vi "Utility Timestamp.vi"() -> (3 "Timestamp String":string)   [LabVIEW 2015]
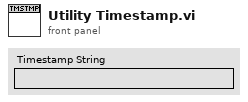
[diagram p1: front panel]
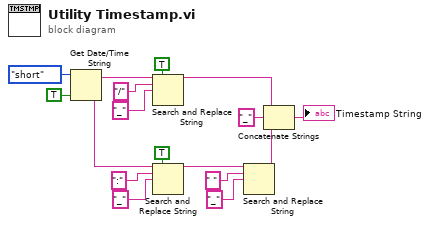
[diagram p0: block diagram]
diagram:
  n1 = Get Date/Time String(date format (0)=enum16{"short", "long", "abbreviated"}."short", want seconds? (F)=TRUE) -> (date string=w15:string, time string=w2:string)  [unwired: 1 in]
  n2 = Search and Replace String(replace all?=TRUE ("replace all? (F)"), input string=w15, search string="/", replace string="_" ("replace string (\"\")")) -> (result string=w1:string)  [unwired: 4 in, 3 out]
  n3 = Search and Replace String(replace all?=TRUE ("replace all? (F)"), input string=w2, search string=":", replace string="_" ("replace string (\"\")")) -> (result string=w6:string)  [unwired: 4 in, 3 out]
  n4 = Search and Replace String(input string=w6, search string=" ", replace string="_" ("replace string (\"\")")) -> (result string=w3:string)  [unwired: 5 in, 3 out]
  n5 = Concatenate Strings(w1, "_" ("string"), w3) -> (→"Timestamp String":string)
